vi "Motor conditions_L298.vi"(6 "error in (no error)":errorcluster, 8 "Angle Tolerance":dbl=0.2 min=0.2, 9 "stop":bool, 10 "Target Angle (-90to90)":dbl, 11 "Start Location Step (-90to90)":i32) -> (0 "error out":errorcluster, 2 "Waveform Chart":dbl(graph), 3 "Current Motor Step (0to3)":i32)   [LabVIEW 2017]
uses:
  <vilib>/myRIO/Instrument Drivers/Onboard IO/DIO/typedefs/DIO Reference.ctl
  <vilib>/myRIO/Common/Instrument Driver Framework/Utilities/typedefs/myRIO Generic Hardware Reference.ctl
  <vilib>/myRIO/Common/Instrument Driver Framework/Utilities/typedefs/Hardware Version Enum.ctl
  <vilib>/myRIO/Common/Instrument Driver Framework/Utilities/typedefs/myRIO v1.0 Reference.ctl
  <vilib>/myRIO/Common/Instrument Driver Framework/Utilities/typedefs/Generic FPGA Reference.ctl
  <vilib>/myRIO/Common/Instrument Driver Framework/myRIO v1.0/DIO/typedefs/DIO Channels List.ctl
  <vilib>/myRIO/Common/Instrument Driver Framework/myRIO v1.0/DIO/typedefs/DIO Channels Enum.ctl
  <vilib>/userdefined/High Color/nirio_resource_hc.ctl
  <vilib>/myRIO/Instrument Drivers/Onboard IO/AI/typedefs/AI Reference.ctl
  <vilib>/myRIO/Common/Instrument Driver Framework/myRIO v1.0/AI/typedefs/AI Channels List.ctl
  <vilib>/myRIO/Common/Instrument Driver Framework/myRIO v1.0/AI/typedefs/AI Channels Enum.ctl
  <vilib>/myRIO/Common/Instrument Driver Framework/Utilities/typedefs/Analog Scaling Constants List.ctl
  <vilib>/myRIO/Common/Instrument Driver Framework/Utilities/typedefs/Analog Scaling Constants.ctl
  <vilib>/myRIO/Common/Instrument Driver Framework/Utilities/vis/Is FPGA Ref Available.vi
  <vilib>/myRIO/Common/Instrument Driver Framework/myRIO v1.0/DIO/vis/myRIO v1.1 Open DIO.vi
  <vilib>/myRIO/Instrument Drivers/Onboard IO/DIO/vis/Write.vi
  <vilib>/myRIO/Common/Instrument Driver Framework/myRIO v1.0/AI/vis/myRIO v1.1 Open AI.vi
  <vilib>/myRIO/Instrument Drivers/Onboard IO/AI/vis/Read.vi
  <vilib>/myRIO/Common/Instrument Driver Framework/Utilities/vis/Validate Channels.vi
  <vilib>/myRIO/Common/Instrument Driver Framework/myRIO v1.0/DIO/vis/myRIO v1.0 Reserve DIO.vi
  <vilib>/myRIO/Common/Instrument Driver Framework/myRIO v1.0/AI/vis/myRIO v1.0 Reserve AI.vi
  <vilib>/myRIO/Common/Instrument Driver Framework/myRIO v1.0/Resource Manager/vis/myRIO v1.0 Reserve Channel List.vi
  <vilib>/myRIO/Common/Instrument Driver Framework/myRIO v1.0/DIO/vis/myRIO v1.0 Build MUX Configuration DIO.vi
  <vilib>/myRIO/Common/Instrument Driver Framework/myRIO v1.0/AI/vis/myRIO v1.0 Build MUX Configuration AI.vi
  <vilib>/myRIO/Common/Instrument Driver Framework/myRIO v1.0/Resource Manager/vis/myRIO v1.0 Reserve Channel.vi
  <vilib>/myRIO/Common/Instrument Driver Framework/myRIO v1.0/Resource Manager/vis/myRIO v1.0 Unreserve Channel.vi
  <vilib>/myRIO/Common/Instrument Driver Framework/myRIO v1.0/Resource Manager/vis/myRIO v1.0 Create Configuration List.vi
  <vilib>/myRIO/Common/Instrument Driver Framework/myRIO v1.0/Resource Manager/vis/myRIO v1.0 Build Mutex Name.vi
  <vilib>/Utility/VariantDataType/GetNumericInfo.vi
  <vilib>/Utility/error.llb/Error Cluster From Error Code.vi
  <vilib>/myRIO/Common/Instrument Driver Framework/myRIO v1.0/myRIO v1.1 Open.vi
  <vilib>/myRIO/Common/Instrument Driver Framework/myRIO v1.0/AI/vis/myRIO v1.0 Get Scaling Constants AI.vi
  <vilib>/myRIO/Common/Instrument Driver Framework/Utilities/vis/IO Manager.vi
  <vilib>/myRIO/Common/Instrument Driver Framework/Utilities/vis/Configuration Manager.vi
  <vilib>/myRIO/Common/Instrument Driver Framework/myRIO v1.0/myRIO v1.0 Close.vi
  <vilib>/myRIO/Common/Instrument Driver Framework/myRIO v1.0/AI/vis/myRIO v1.0 Read AI.vi
  <vilib>/myRIO/Common/Instrument Driver Framework/myRIO v1.0/Resource Manager/vis/myRIO v1.0 Configure IO.vi
  <vilib>/myRIO/Common/Instrument Driver Framework/myRIO v1.0/DIO/vis/myRIO v1.0 Write DIO.vi
  <vilib>/myRIO/Express VI/Onboard IO/AI/AI Express VI.xnode
  <vilib>/myRIO/Instrument Drivers/Onboard IO/AI/vis/myRIO AI Open.xnode
  <vilib>/myRIO/Express VI/Onboard IO/DO/DO Express VI.xnode
  <vilib>/myRIO/Instrument Drivers/Onboard IO/DIO/vis/myRIO DIO Open.xnode
  <vilib>/myRIO/Instrument Drivers/Onboard IO/DIO/DIO.lvlib
  <vilib>/myRIO/Instrument Drivers/Onboard IO/AI/AI.lvlib
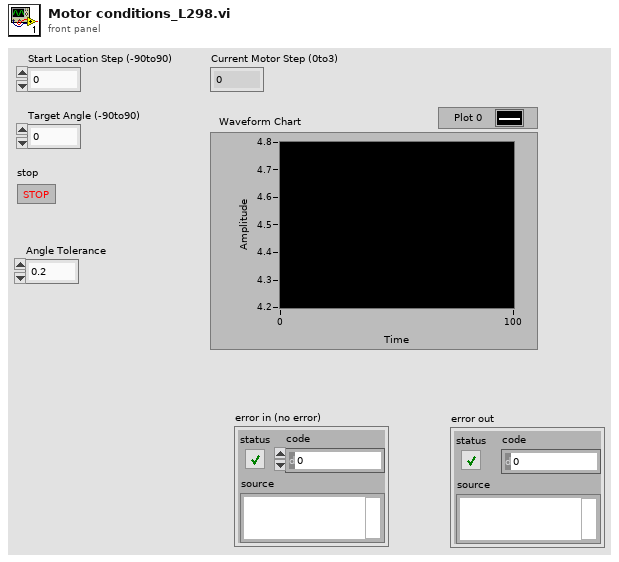
[diagram p1: front panel]
types:
  T1 = typedef "AI.lvlib/AI Reference.ctl" = cluster{"myRIO Reference":T2, "AI Channels List":T6, "AI Scaling Constants List":T8}
  T2 = typedef "myRIO Generic Hardware Reference.ctl" = cluster{"myRIO Model":T3, "myRIO Hardware Reference":T4}
  T3 = typedef "Hardware Version Enum.ctl" = enum16{"Unknown", "myRIO-1900", "myRIO-1950", "roboRIO", "NI ELVIS RIO CM"}
  T4 = typedef "myRIO v1.0 Reference.ctl" = cluster{"Generic FPGA Reference":T5, "Allow multiple opens":bool}
  T5 = typedef "Generic FPGA Reference.ctl" = refnum<k20>
  T6 = typedef "AI Channels List.ctl" = T7[]
  T7 = typedef "AI Channels Enum.ctl" = enum16{"Not Connected", "AudioIn/Left", "AudioIn/Right", "C/AI0", "C/AI1", "A/AI0", "A/AI1", "A/AI2", "A/AI3", "B/AI0", "B/AI1", "B/AI2", "B/AI3", "AI/AI0", "AI/AI1", "AI/AI2", "AI/AI3"}
  T8 = typedef "Analog Scaling Constants List.ctl" = T9[]
  T9 = typedef "Analog Scaling Constants.ctl" = cluster{"LSB Weight (Volts)":dbl, "Offset (Volts)":dbl, "Signed?":bool}
  T10 = typedef "nirio_resource_hc.ctl" = tag
  T11 = typedef "DIO.lvlib/DIO Reference.ctl" = cluster{"myRIO Reference":T2, "DIO Channels List":T12}
  T12 = typedef "DIO Channels List.ctl" = T13[]
  T13 = typedef "DIO Channels Enum.ctl" = enum16{"Not Connected", "C/DIO0", "C/DIO1", "C/DIO2", "C/DIO3", "C/DIO4", "C/DIO5", "C/DIO6", "C/DIO7", "A/DIO0", "A/DIO1", "A/DIO2", "A/DIO3", "A/DIO4", "A/DIO5", "A/DIO6", "A/DIO7", "A/DIO8", "A/DIO9", "A/DIO10", "A/DIO11", "A/DIO12", "A/DIO13", "A/DIO14", "A/DIO15", "B/DIO0", "B/DIO1", "B/DIO2", "B/DIO3", "B/DIO4", "B/DIO5", "B/DIO6", "B/DIO7", "B/DIO8", "B/DIO9", "B/DIO10", "B/DIO11", "B/DIO12", "B/DIO13", "B/DIO14", "B/DIO15", "LED0", "LED1", "LED2", "LED3", "Button0", "DIO/DIO0", "DIO/DIO1", "DIO/DIO2", "DIO/DIO3", "DIO/DIO4", "DIO/DIO5", "DIO/DIO6", "DIO/DIO7", "DIO/DIO8", "DIO/DIO9", "SPI/CS0", "SPI/CS1", "SPI/CS2", "SPI/CS3", "LED RADIO (Green)", "LED RADIO (Red)", "LED COMM (Green)", "LED COMM (Red)", "LED MODE (Green)", "LED MODE (Red)"}
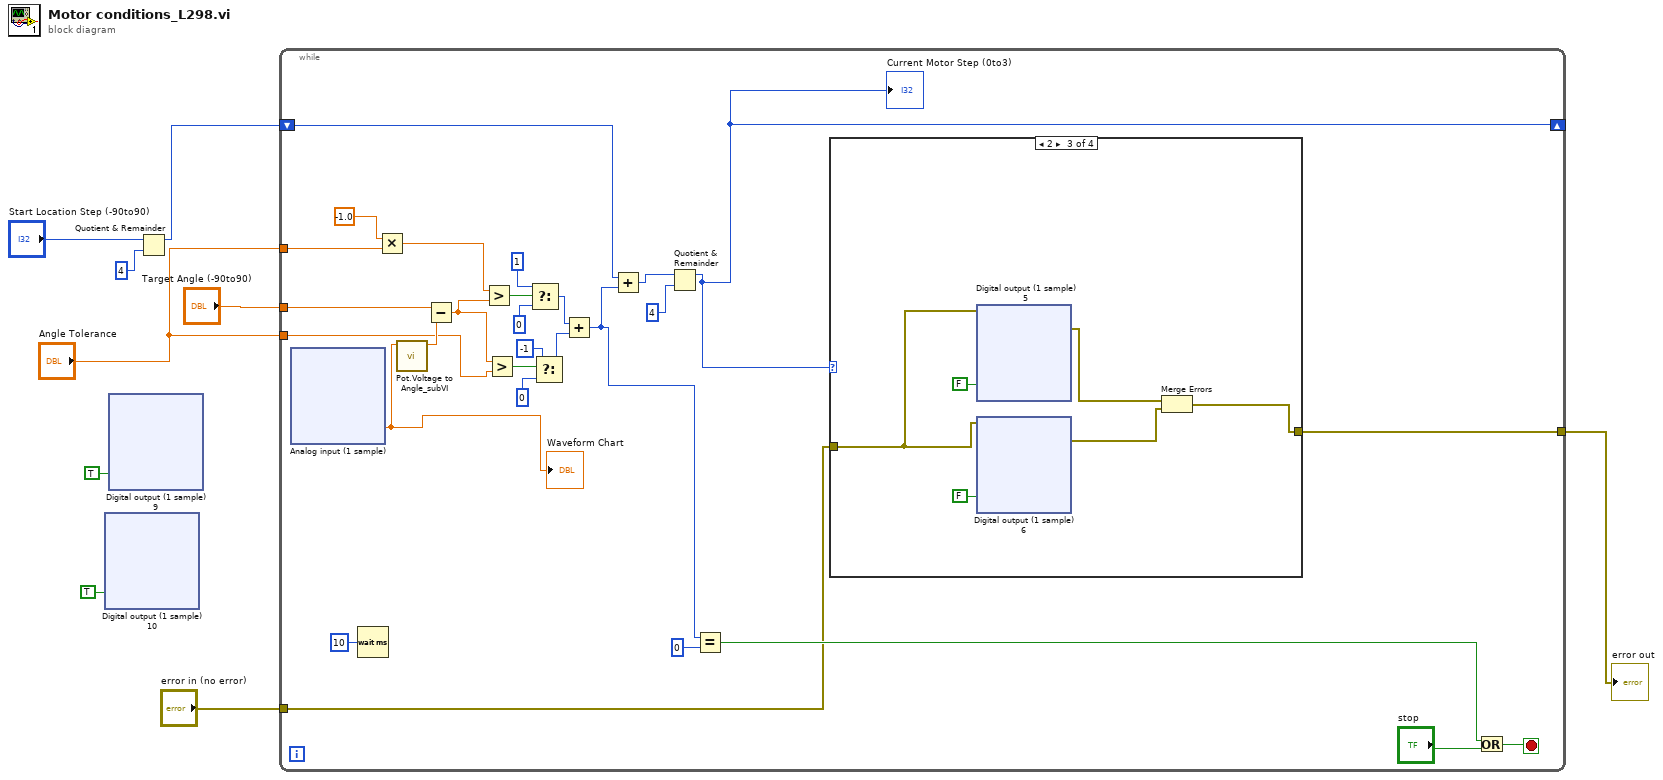
[diagram p0: block diagram]
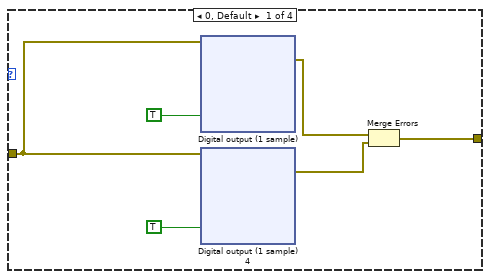
[diagram p2: hidden frame]
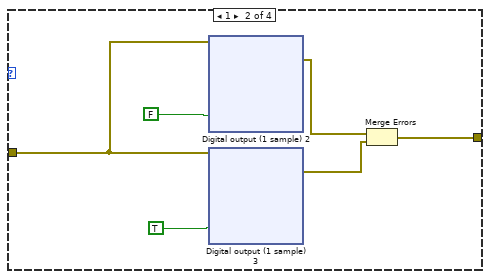
[diagram p3: hidden frame]
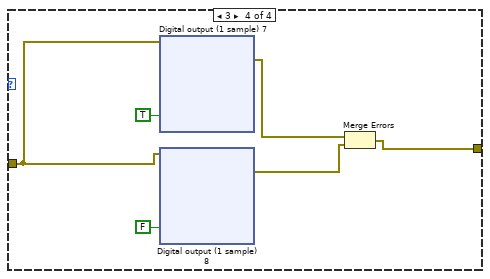
[diagram p4: hidden frame]
diagram:
  n1 = xnode "Digital output (1 sample) 10"("C/DIO3 (DIO3)"=TRUE) -> ()  [unwired: 1 in, 1 out]
  n2 = xnode "Digital output (1 sample) 9"("A/DIO10 (Pin 31)"=TRUE) -> ()  [unwired: 1 in, 1 out]
  n3 = Quotient & Remainder(x="Start Location Step (-90to90)", y=4) -> (x-y*floor(x/y)=w7:i32)  [unwired: 1 out]
  n4 = while {
    tunnel: "Target Angle (-90to90)" -> [w24]
    shift-right: [w25] -> _
    shift-left: w7 -> [w26]
    tunnel: "Angle Tolerance" -> [w13]
    tunnel: "Angle Tolerance" -> [w12]
    tunnel: "error in (no error)" -> [w11]
    tunnel: [w10] -> w1
    stop <- w23 stop-if-true
    n5 = xnode "Analog input (1 sample)"() -> ("A/AI2 (Pin 7)"=w16:dbl)  [unwired: 1 in, 1 out]
    "Waveform Chart" <- w16
    n6 = Wait (ms)(milliseconds to wait=u32 10) -> ()  [unwired: 1 out]
    n7 = Multiply(x=-1.0, y=w13) -> (x*y=w14:dbl)
    n8 = call "Pot.Voltage to Angle_subVI.vi"("Potentiometer V (0-5)"=w16) -> ("Pull-back angle (°)"=w17:dbl)  [unwired: 10 in]
    n9 = Subtract(x=w24, y=w17) -> (x-y=w37:dbl)
    n10 = Greater?(x=w14, y=w37) -> (0:w36:bool)
    n11 = Greater?(x=w37, y=w12) -> (0:w33:bool)
    n12 = Select(t=1, s=w36, f=0) -> (s? t:f=w30:i32)
    n13 = Select(t=-1, s=w33, f=0) -> (s? t:f=w29:i32)
    n14 = Add(x=w30, y=w29) -> (x+y=w20:i32)
    n15 = Add(x=w26, y=w20) -> (x+y=w28:i32)
    n16 = Quotient & Remainder(x=w28, y=4) -> (x-y*floor(x/y)=w25:i32)  [unwired: 1 out]
    "Current Motor Step (0to3)" <- w25
    n17 = Equal?(x=w20, y=0) -> (x = y?=w21:bool)
    n18 = case shown="2" w25 {
      tunnel: w11 -> [w78 w154 w230 w306]
      tunnel: [w75 w151 w227 w303] -> w10
      frame 0, Default {
        n19 = xnode "Digital output (1 sample)"("C/DIO5 (DIO5)"=TRUE, "error in (no error)"=w78) -> ("error out"=w77:errorcluster)
        n20 = xnode "Digital output (1 sample) 4"("C/DIO4 (DIO4)"=TRUE, "error in (no error)"=w78) -> ("error out"=w76:errorcluster)
        n21 = Merge Errors(w77, w76) -> (w75:errorcluster)
      }
      frame 1 {
        n22 = xnode "Digital output (1 sample) 2"("C/DIO5 (DIO5)"=FALSE, "error in (no error)"=w154) -> ("error out"=w153:errorcluster)
        n23 = xnode "Digital output (1 sample) 3"("C/DIO4 (DIO4)"=TRUE, "error in (no error)"=w154) -> ("error out"=w152:errorcluster)
        n24 = Merge Errors(w153, w152) -> (w151:errorcluster)
      }
      frame 2 {
        n25 = xnode "Digital output (1 sample) 5"("C/DIO5 (DIO5)"=FALSE, "error in (no error)"=w230) -> ("error out"=w229:errorcluster)
        n26 = xnode "Digital output (1 sample) 6"("C/DIO4 (DIO4)"=FALSE, "error in (no error)"=w230) -> ("error out"=w228:errorcluster)
        n27 = Merge Errors(w229, w228) -> (w227:errorcluster)
      }
      frame 3 {
        n28 = xnode "Digital output (1 sample) 7"("C/DIO5 (DIO5)"=TRUE, "error in (no error)"=w306) -> ("error out"=w305:errorcluster)
        n29 = xnode "Digital output (1 sample) 8"("C/DIO4 (DIO4)"=FALSE, "error in (no error)"=w306) -> ("error out"=w304:errorcluster)
        n30 = Merge Errors(w305, w304) -> (w303:errorcluster)
      }
    }
    n31 = Or(x=w21, y="stop") -> (x .or. y?=w23:bool)
  }
  "error out" <- w1
